vi "get_amp_phas.vi"(8 "error in (no error)":errorcluster, 11 "Lock-In Amplifier in":refnum<class "Lock-In Amplifier.lvclass">) -> (0 "error out":errorcluster, 1 "Phase (rad)":dbl, 2 "Amplitude (V rms)":dbl, 3 "Lock-In Amplifier out":refnum<class "Lock-In Amplifier.lvclass">)   [LabVIEW 2020, in "Lock-In Amplifier.lvclass"]
uses:
  Lock-In Amplifier.lvclass
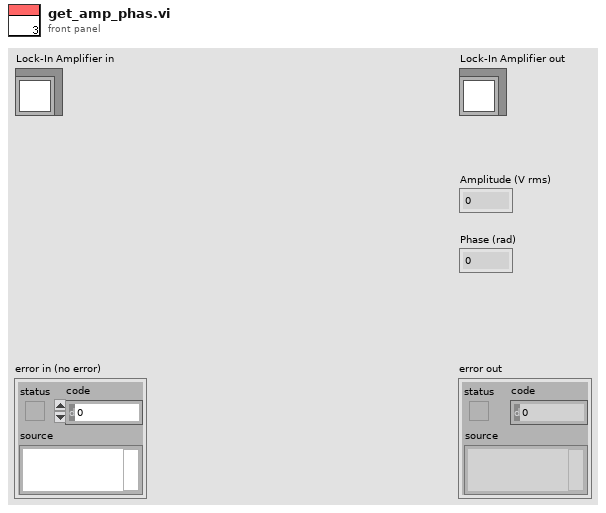
[diagram p1: front panel]
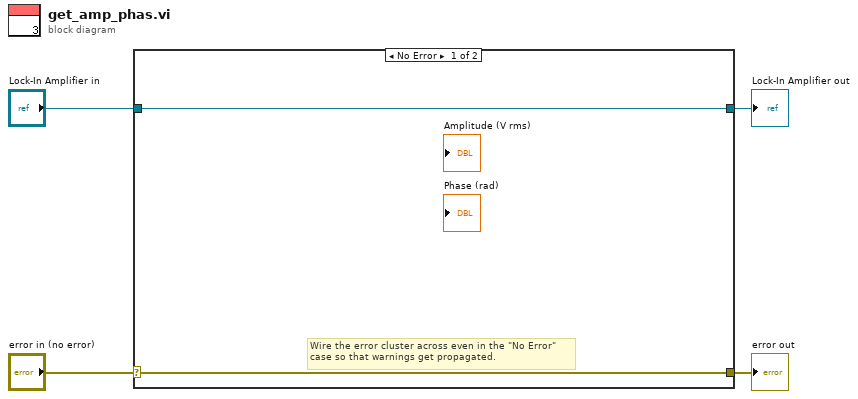
[diagram p0: block diagram]
diagram:
  n1 = case shown="No Error" "error in (no error)" {
    selector: "error in (no error)" -> [w5 w8]
    tunnel: [w5 w8] -> w3
    tunnel: [w6 w7] -> w1
    tunnel: "Lock-In Amplifier in" -> [w6 w7]
    frame No Error {
      # "Wire the error cluster across even in the \"No Error\"\ncase so that warnings get propagated."
    }
    frame Error {
    }
  }
  "error out" <- w3
  "Lock-In Amplifier out" <- w1
